vi "Toolkit - Is Cluster.vi"() -> ()   [LabVIEW 2017]
doc: "Finds all of the clusters in the block diagram and front panel of a VI using VI scripting and the ACE Toolkit API."
uses:
  <vilib>/Utility/traverseref.llb/TRef TravTarget.ctl
  <vilib>/Utility/traverseref.llb/VI Scripting - Traverse.lvlib
  Toolkit/Toolkit.lvlib
panel:
  out "Block Diagram Object is a Cluster":bool
  out "Front Panel Object is a Cluster":bool
  # "Overview: Demonstrates finding all clusters in a VI using VI scripting the ACE toolkit\nInstructions:\n1. Run this VI"
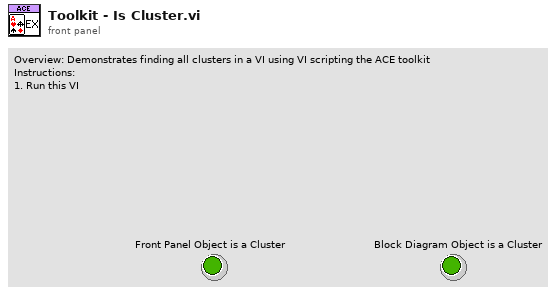
[diagram p1: front panel]
types:
  T1 = typedef "TRef TravTarget.ctl" = enum16{"FP", "BD", "Other"}
  T2 = enum32{"Invalid", "Standard", "Closed", "Hidden", "Minimized", "Maximized"}
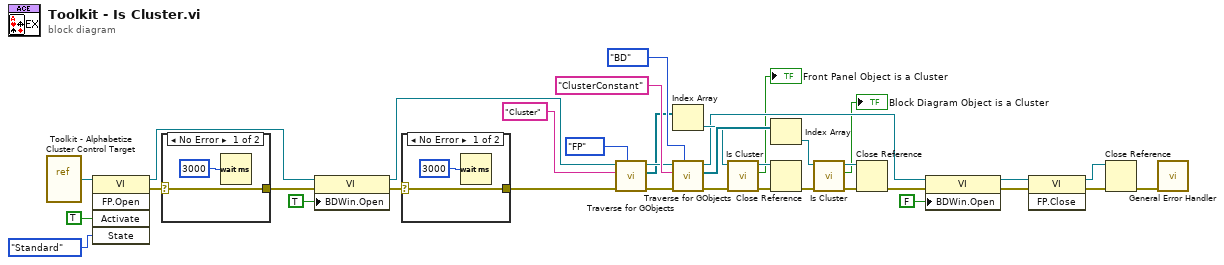
[diagram p0: block diagram]
diagram:
  n1 = vi-ref "Toolkit - Alphabetize Cluster Control Target.vi"() -> (w29:refnum<vi>)
  n2 = invoke class="VI" method="FP.Open"(reference=w29, "Activate"=TRUE ("Activate?"), "State"=T2."Standard") -> (reference out=w31:refnum<vi>, error out=w24:errorcluster)  [unwired: 2 in, 3 out]
  n3 = case shown="No Error" w24 {
    selector: w24 -> [w38 w39]
    tunnel: [w38 w39] -> w23
    frame No Error {
      n4 = Wait (ms)(milliseconds to wait=u32 3000) -> ()  [unwired: 1 out]
    }
    frame Error {
    }
  }
  n5 = property class="VI"(reference=w31, error in=w23, "BDWin.Open"=TRUE ("Block Diagram Window:Open")) -> (reference out=w20:refnum<vi>, error out=w30:errorcluster)
  n6 = case shown="No Error" w30 {
    selector: w30 -> [w41 w42]
    tunnel: [w41 w42] -> w21
    frame No Error {
      n7 = Wait (ms)(milliseconds to wait=u32 3000) -> ()  [unwired: 1 out]
    }
    frame Error {
    }
  }
  n8 = call <vilib>:"Traverse for GObjects.vi"("Traverse Target"=TRef_TravTarget."FP", "error in (no error)"=w21, "Class Name"="Cluster", "VI Refnum"=w20) -> ("error out"=w14:errorcluster, "References"=w13:refnum<vi>[], "dup VI Refnum"=w15:refnum<vi>)  [unwired: 4 in, 1 out]
  n9 = Index Array(array=w13) -> (element=w10:refnum<vi>)  [unwired: 1 in]
  n10 = call <vilib>:"Traverse for GObjects.vi"("Traverse Target"=TRef_TravTarget."BD", "error in (no error)"=w14, "Class Name"="ClusterConstant", "VI Refnum"=w15) -> ("error out"=w11:errorcluster, "References"=w12:refnum<vi>[], "dup VI Refnum"=w3:refnum<vi>)  [unwired: 4 in, 1 out]
  n11 = call "Is Cluster.vi"("Error In"=w11, "GObject In"=w10) -> ("Error Out"=w8:errorcluster, "Cluster?"=→"Front Panel Object is a Cluster":bool, "GObject Out"=w9:refnum<vi>)  [unwired: 7 in]
  n12 = Index Array(array=w12) -> (element=w6:refnum<vi>)  [unwired: 1 in]
  n13 = Close Reference(reference=w9, error in (no error)=w8) -> (error out=w7:errorcluster)
  n14 = call "Is Cluster.vi"("Error In"=w7, "GObject In"=w6) -> ("Error Out"=w4:errorcluster, "Cluster?"=→"Block Diagram Object is a Cluster":bool, "GObject Out"=w5:refnum<vi>)  [unwired: 7 in]
  n15 = Close Reference(reference=w5, error in (no error)=w4) -> (error out=w22:errorcluster)
  n16 = property class="VI"(reference=w3, error in=w22, "BDWin.Open"=FALSE ("Block Diagram Window:Open")) -> (reference out=w27:refnum<vi>, error out=w26:errorcluster)
  n17 = invoke class="VI" method="FP.Close"(reference=w27, error in=w26) -> (reference out=w33:refnum<vi>, error out=w32:errorcluster)  [unwired: 1 in, 1 out]
  n18 = Close Reference(reference=w33, error in (no error)=w32) -> (error out=w36:errorcluster)
  n19 = call <vilib>:"General Error Handler.vi"("error in (no error)"=w36) -> ()  [unwired: 10 in, 5 out]
